vi "VI Tree.vi"   [LabVIEW 2011, in "Fluke 5XXX Series Multicalibrators.lvlib"]
doc: "This is the instrument driver for the following instruments FLUKE 5500A, 5520A, 5700A, 5720A and 57LFC including their options:\n\n 5725A ... Auxiliary amplifier\n SC300 ... 300 MHz Oscilloscope Calibration\n SC600 ... 600 MHz Oscilloscope Calibration\n SC1100 ... 1.1 GHz Oscilloscope Calibration\n 700P ... Pressure modules\n 5700A_03 ... Wideband AC Voltage\n\nThe VI Tree displays all the user-callable VIs of the instrument driver in an organized table."
uses:
  Fluke 5XXX Series Multicalibrators.lvlib
panel:
  # "© 2005 National Instruments.  ALL RIGHTS RESERVED."
  # "SEE DIAGRAM\nFOR VI TREE."
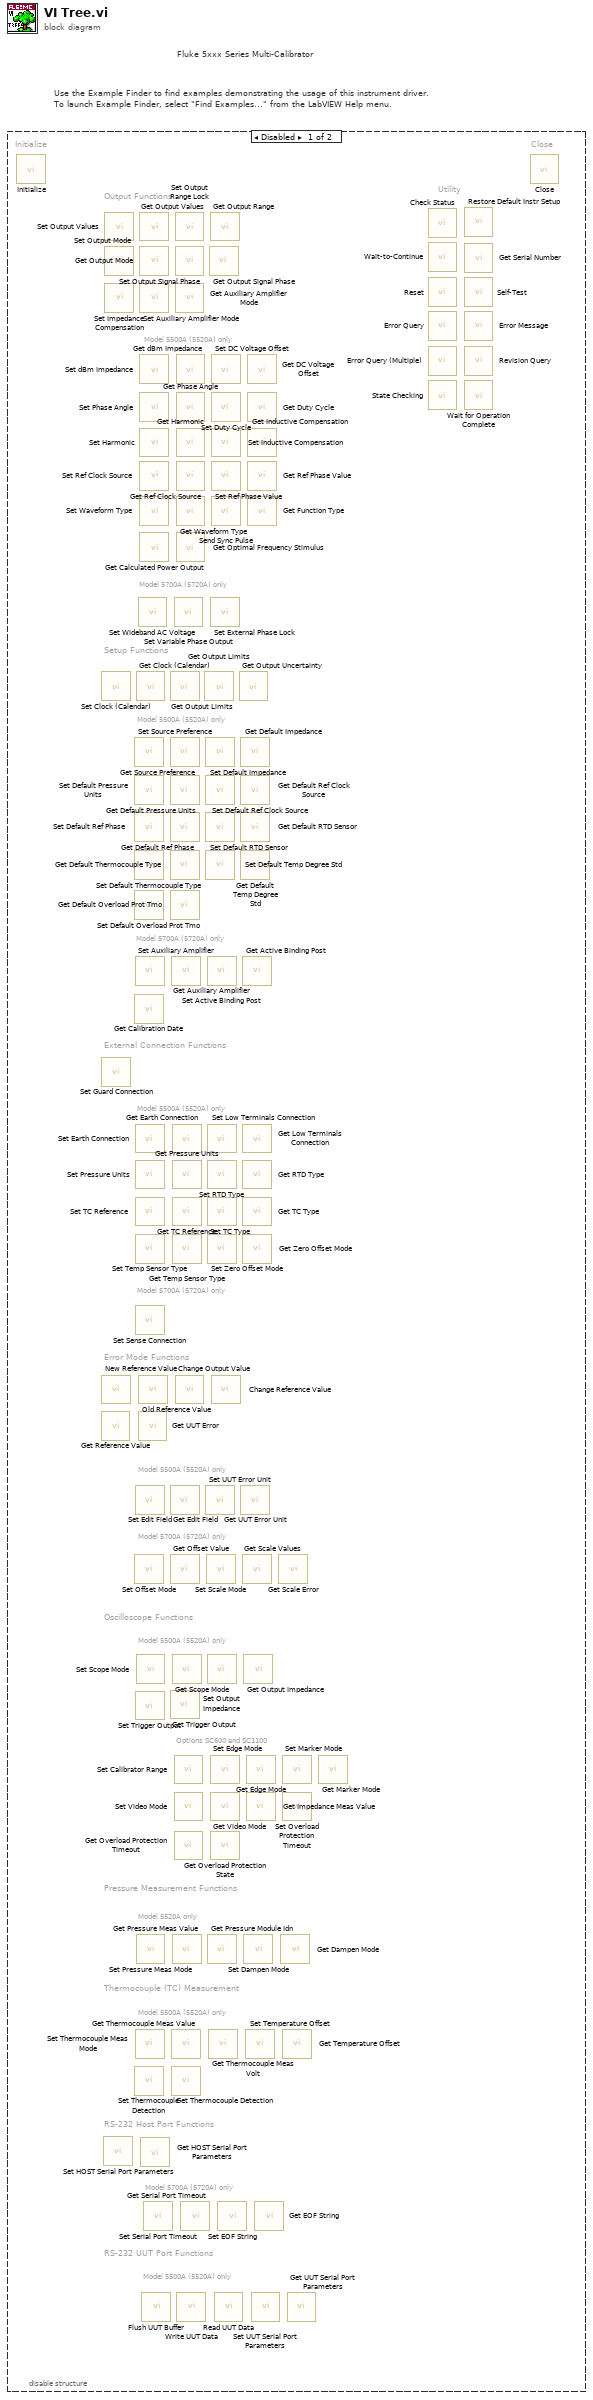
[diagram p0: block diagram]
diagram:
  # "Fluke 5xxx Series Multi-Calibrator"
  # "Use the Example Finder to find examples demonstrating the usage of this instrument driver.\nTo launch Example Finder, select \"Find Examples...\" from the LabVIEW Help menu."
  n1 = disable-structure shown="Disabled" {
    frame Disabled {
      # "Model 5500A (5520A) only"
      # "RS-232 UUT Port Functions"
      # "Model 5700A (5720A) only"
      # "RS-232 Host Port Functions"
      # "Model 5500A (5520A) only"
      # "Thermocouple (TC) Measurement"
      # "Model 5520A only"
      # "Pressure Measurement Functions"
      # "Options SC600 and SC1100"
      # "Model 5500A (5520A) only"
      # "Oscilloscope Functions"
      # "Model 5700A (5720A) only"
      # "Model 5500A (5520A) only"
      # "Error Mode Functions"
      # "Model 5700A (5720A) only"
      # "Model 5500A (5520A) only"
      # "External Connection Functions"
      # "Model 5700A (5720A) only"
      # "Model 5500A (5520A) only"
      # "Setup Functions"
      # "Model 5700A (5720A) only"
      # "Model 5500A (5520A) only"
      # "Output Functions"
      # "Utility"
      # "Close"
      # "Initialize"
      n2 = call "Initialize.vi"() -> ()  [unwired: 14 in, 2 out]
      n3 = call "Get Reference Value.vi"() -> ()  [unwired: 9 in, 3 out]
      n4 = call "Set Clock (Calendar).vi"() -> ()  [unwired: 14 in, 2 out]
      n5 = call "Set Guard Connection.vi"() -> ()  [unwired: 10 in, 2 out]
      n6 = call "New Reference Value.vi"() -> ()  [unwired: 10 in, 2 out]
      n7 = call "Set HOST Serial Port Parameters.vi"() -> ()  [unwired: 14 in, 2 out]
      n8 = call "Set Output Values.vi"() -> ()  [unwired: 10 in, 2 out]
      n9 = call "Set Output Mode.vi"() -> ()  [unwired: 10 in, 2 out]
      n10 = call "Set Impedance Compensation.vi"() -> ()  [unwired: 10 in, 2 out]
      n11 = call "Set Source Preference.vi"() -> ()  [unwired: 10 in, 2 out]
      n12 = call "Set Default Pressure Units.vi"() -> ()  [unwired: 10 in, 2 out]
      n13 = call "Set Default Ref Phase.vi"() -> ()  [unwired: 10 in, 2 out]
      n14 = call "Set Default Thermocouple Type.vi"() -> ()  [unwired: 10 in, 2 out]
      n15 = call "Set Default Overload Prot Tmo.vi"() -> ()  [unwired: 10 in, 2 out]
      n16 = call "Get Calibration Date.vi"() -> ()  [unwired: 7 in, 5 out]
      n17 = call "Set Offset Mode.vi"() -> ()  [unwired: 10 in, 2 out]
      n18 = call "Set Thermocouple Detection.vi"() -> ()  [unwired: 10 in, 2 out]
      n19 = call "Set Auxiliary Amplifier.vi"() -> ()  [unwired: 10 in, 2 out]
      n20 = call "Set Earth Connection.vi"() -> ()  [unwired: 10 in, 2 out]
      n21 = call "Set Pressure Units.vi"() -> ()  [unwired: 10 in, 2 out]
      n22 = call "Set TC Reference.vi"() -> ()  [unwired: 10 in, 2 out]
      n23 = call "Set Temp Sensor Type.vi"() -> ()  [unwired: 10 in, 2 out]
      n24 = call "Set Sense Connection.vi"() -> ()  [unwired: 10 in, 2 out]
      n25 = call "Set Edit Field.vi"() -> ()  [unwired: 10 in, 2 out]
      n26 = call "Set Trigger Output.vi"() -> ()  [unwired: 10 in, 2 out]
      n27 = call "Set Thermocouple Meas Mode.vi"() -> ()  [unwired: 10 in, 2 out]
      n28 = call "Get Clock (Calendar).vi"() -> ()  [unwired: 8 in, 8 out]
      n29 = call "Set Scope Mode.vi"() -> ()  [unwired: 10 in, 2 out]
      n30 = call "Set Pressure Meas Mode.vi"() -> ()  [unwired: 10 in, 2 out]
      n31 = call "Set Wideband AC Voltage.vi"() -> ()  [unwired: 10 in, 2 out]
      n32 = call "Get UUT Error.vi"() -> ()  [unwired: 8 in, 4 out]
      n33 = call "Old Reference Value.vi"() -> ()  [unwired: 10 in, 2 out]
      n34 = call "Get Output Values.vi"() -> ()  [unwired: 9 in, 7 out]
      n35 = call "Get Output Mode.vi"() -> ()  [unwired: 9 in, 3 out]
      n36 = call "Set Auxiliary Amplifier Mode.vi"() -> ()  [unwired: 10 in, 2 out]
      n37 = call "Set dBm Impedance.vi"() -> ()  [unwired: 10 in, 2 out]
      n38 = call "Set Phase Angle.vi"() -> ()  [unwired: 10 in, 2 out]
      n39 = call "Set Harmonic.vi"() -> ()  [unwired: 10 in, 2 out]
      n40 = call "Set Ref Clock Source.vi"() -> ()  [unwired: 10 in, 2 out]
      n41 = call "Set Waveform Type.vi"() -> ()  [unwired: 10 in, 2 out]
      n42 = call "Get Calculated Power Output.vi"() -> ()  [unwired: 9 in, 3 out]
      n43 = call "Get HOST Serial Port Parameters.vi"() -> ()  [unwired: 7 in, 9 out]
      n44 = call "Flush UUT Buffer.vi"() -> ()  [unwired: 10 in, 2 out]
      n45 = call "Set Serial Port Timeout.vi"() -> ()  [unwired: 10 in, 2 out]
      n46 = call "Get Output Limits.vi"() -> ()  [unwired: 8 in, 4 out]
      n47 = call "Get Source Preference.vi"() -> ()  [unwired: 9 in, 3 out]
      n48 = call "Get Default Pressure Units.vi"() -> ()  [unwired: 9 in, 3 out]
      n49 = call "Get Default Ref Phase.vi"() -> ()  [unwired: 9 in, 3 out]
      n50 = call "Get Default Thermocouple Type.vi"() -> ()  [unwired: 9 in, 3 out]
      n51 = call "Get Default Overload Prot Tmo.vi"() -> ()  [unwired: 9 in, 3 out]
      n52 = call "Get Edit Field.vi"() -> ()  [unwired: 9 in, 3 out]
      n53 = call "Get Offset Value.vi"() -> ()  [unwired: 8 in, 4 out]
      n54 = call "Get Trigger Output.vi"() -> ()  [unwired: 9 in, 3 out]
      n55 = call "Get Auxiliary Amplifier.vi"() -> ()  [unwired: 8 in, 4 out]
      n56 = call "Get Thermocouple Meas Value.vi"() -> ()  [unwired: 8 in, 4 out]
      n57 = call "Get Thermocouple Detection.vi"() -> ()  [unwired: 9 in, 3 out]
      n58 = call "Get Earth Connection.vi"() -> ()  [unwired: 9 in, 3 out]
      n59 = call "Get Pressure Units.vi"() -> ()  [unwired: 9 in, 3 out]
      n60 = call "Get TC Reference.vi"() -> ()  [unwired: 7 in, 5 out]
      n61 = call "Get Temp Sensor Type.vi"() -> ()  [unwired: 9 in, 3 out]
      n62 = call "Get Scope Mode.vi"() -> ()  [unwired: 9 in, 3 out]
      n63 = call "Get Pressure Meas Value.vi"() -> ()  [unwired: 8 in, 4 out]
      n64 = call "Set Variable Phase Output.vi"() -> ()  [unwired: 10 in, 2 out]
      n65 = call "Set Calibrator Range.vi"() -> ()  [unwired: 10 in, 2 out]
      n66 = call "Set Video Mode.vi"() -> ()  [unwired: 10 in, 2 out]
      n67 = call "Get Overload Protection Timeout.vi"() -> ()  [unwired: 9 in, 3 out]
      n68 = call "Set Output Range Lock.vi"() -> ()  [unwired: 10 in, 2 out]
      n69 = call "Set Output Signal Phase.vi"() -> ()  [unwired: 10 in, 2 out]
      n70 = call "Get Auxiliary Amplifier Mode.vi"() -> ()  [unwired: 9 in, 3 out]
      n71 = call "Change Output Value.vi"() -> ()  [unwired: 10 in, 2 out]
      n72 = call "Get dBm Impedance.vi"() -> ()  [unwired: 9 in, 3 out]
      n73 = call "Get Phase Angle.vi"() -> ()  [unwired: 8 in, 4 out]
      n74 = call "Get Harmonic.vi"() -> ()  [unwired: 8 in, 4 out]
      n75 = call "Get Ref Clock Source.vi"() -> ()  [unwired: 9 in, 3 out]
      n76 = call "Get Waveform Type.vi"() -> ()  [unwired: 8 in, 4 out]
      n77 = call "Get Optimal Frequency Stimulus.vi"() -> ()  [unwired: 9 in, 3 out]
      n78 = call "Write UUT Data.vi"() -> ()  [unwired: 10 in, 2 out]
      n79 = call "Get Serial Port Timeout.vi"() -> ()  [unwired: 9 in, 3 out]
      n80 = call "Get Output Limits.vi"() -> ()  [unwired: 8 in, 4 out]
      n81 = call "Set Default Impedance.vi"() -> ()  [unwired: 10 in, 2 out]
      n82 = call "Set Default Ref Clock Source.vi"() -> ()  [unwired: 10 in, 2 out]
      n83 = call "Set Default RTD Sensor.vi"() -> ()  [unwired: 10 in, 2 out]
      n84 = call "Set Default Temp Degree Std.vi"() -> ()  [unwired: 10 in, 2 out]
      n85 = call "Set UUT Error Unit.vi"() -> ()  [unwired: 10 in, 2 out]
      n86 = call "Set Scale Mode.vi"() -> ()  [unwired: 10 in, 2 out]
      n87 = call "Set Active Binding Post.vi"() -> ()  [unwired: 10 in, 2 out]
      n88 = call "Set Low Terminals Connection.vi"() -> ()  [unwired: 10 in, 2 out]
      n89 = call "Set RTD Type.vi"() -> ()  [unwired: 10 in, 2 out]
      n90 = call "Set TC Type.vi"() -> ()  [unwired: 10 in, 2 out]
      n91 = call "Set Zero Offset Mode.vi"() -> ()  [unwired: 10 in, 2 out]
      n92 = call "Set Output Impedance.vi"() -> ()  [unwired: 10 in, 2 out]
      n93 = call "Get Pressure Module Idn.vi"() -> ()  [unwired: 7 in, 5 out]
      n94 = call "Get Thermocouple Meas Volt.vi"() -> ()  [unwired: 9 in, 3 out]
      n95 = call "Get Output Signal Phase.vi"() -> ()  [unwired: 9 in, 3 out]
      n96 = call "Get Output Range.vi"() -> ()  [unwired: 8 in, 4 out]
      n97 = call "Set External Phase Lock.vi"() -> ()  [unwired: 10 in, 2 out]
      n98 = call "Set Edge Mode.vi"() -> ()  [unwired: 10 in, 2 out]
      n99 = call "Get Video Mode.vi"() -> ()  [unwired: 8 in, 4 out]
      n100 = call "Get Overload Protection State.vi"() -> ()  [unwired: 9 in, 3 out]
      n101 = call "Set DC Voltage Offset.vi"() -> ()  [unwired: 10 in, 2 out]
      n102 = call "Set Duty Cycle.vi"() -> ()  [unwired: 10 in, 2 out]
      n103 = call "Set Inductive Compensation.vi"() -> ()  [unwired: 10 in, 2 out]
      n104 = call "Set Ref Phase Value.vi"() -> ()  [unwired: 10 in, 2 out]
      n105 = call "Send Sync Pulse.vi"() -> ()  [unwired: 10 in, 2 out]
      n106 = call "Change Reference Value.vi"() -> ()  [unwired: 10 in, 2 out]
      n107 = call "Read UUT Data.vi"() -> ()  [unwired: 8 in, 4 out]
      n108 = call "Set EOF String.vi"() -> ()  [unwired: 10 in, 2 out]
      n109 = call "Get Output Uncertainty.vi"() -> ()  [unwired: 7 in, 5 out]
      n110 = call "Get Default Impedance.vi"() -> ()  [unwired: 9 in, 3 out]
      n111 = call "Get Default Ref Clock Source.vi"() -> ()  [unwired: 9 in, 3 out]
      n112 = call "Get Default RTD Sensor.vi"() -> ()  [unwired: 9 in, 3 out]
      n113 = call "Get Default Temp Degree Std.vi"() -> ()  [unwired: 9 in, 3 out]
      n114 = call "Get UUT Error Unit.vi"() -> ()  [unwired: 9 in, 3 out]
      n115 = call "Get Active Binding Post.vi"() -> ()  [unwired: 9 in, 3 out]
      n116 = call "Get Low Terminals Connection.vi"() -> ()  [unwired: 9 in, 3 out]
      n117 = call "Get RTD Type.vi"() -> ()  [unwired: 9 in, 3 out]
      n118 = call "Get TC Type.vi"() -> ()  [unwired: 9 in, 3 out]
      n119 = call "Get Zero Offset Mode.vi"() -> ()  [unwired: 7 in, 5 out]
      n120 = call "Get Scale Values.vi"() -> ()  [unwired: 7 in, 5 out]
      n121 = call "Get Output Impedance.vi"() -> ()  [unwired: 9 in, 3 out]
      n122 = call "Set Dampen Mode.vi"() -> ()  [unwired: 10 in, 2 out]
      n123 = call "Set Temperature Offset.vi"() -> ()  [unwired: 10 in, 2 out]
      n124 = call "Get Edge Mode.vi"() -> ()  [unwired: 9 in, 3 out]
      n125 = call "Get Impedance Meas Value.vi"() -> ()  [unwired: 8 in, 4 out]
      n126 = call "Get DC Voltage Offset.vi"() -> ()  [unwired: 9 in, 3 out]
      n127 = call "Get Duty Cycle.vi"() -> ()  [unwired: 9 in, 3 out]
      n128 = call "Get Inductive Compensation.vi"() -> ()  [unwired: 9 in, 3 out]
      n129 = call "Get Ref Phase Value.vi"() -> ()  [unwired: 9 in, 3 out]
      n130 = call "Get Function Type.vi"() -> ()  [unwired: 9 in, 3 out]
      n131 = call "Set UUT Serial Port Parameters.vi"() -> ()  [unwired: 14 in, 2 out]
      n132 = call "Get EOF String.vi"() -> ()  [unwired: 8 in, 4 out]
      n133 = call "Get Scale Error.vi"() -> ()  [unwired: 8 in, 4 out]
      n134 = call "Get Dampen Mode.vi"() -> ()  [unwired: 9 in, 3 out]
      n135 = call "Set Marker Mode.vi"() -> ()  [unwired: 10 in, 2 out]
      n136 = call "Set Overload Protection Timeout.vi"() -> ()  [unwired: 10 in, 2 out]
      n137 = call "Get Temperature Offset.vi"() -> ()  [unwired: 8 in, 4 out]
      n138 = call "Get UUT Serial Port Parameters.vi"() -> ()  [unwired: 9 in, 7 out]
      n139 = call "Get Marker Mode.vi"() -> ()  [unwired: 9 in, 3 out]
      n140 = call "Check Status.vi"() -> ()  [unwired: 14 in, 2 out]
      n141 = call "Wait-to-Continue.vi"() -> ()  [unwired: 10 in, 2 out]
      n142 = call "Reset.vi"() -> ()  [unwired: 14 in, 2 out]
      n143 = call "Error Query.vi"() -> ()  [unwired: 12 in, 4 out]
      n144 = call "Error Query (Multiple).vi"() -> ()  [unwired: 12 in, 4 out]
      n145 = call "State Checking.vi"() -> ()  [unwired: 10 in, 2 out]
      n146 = call "Restore Default Instr Setup.vi"() -> ()  [unwired: 10 in, 2 out]
      n147 = call "Get Serial Number.vi"() -> ()  [unwired: 9 in, 3 out]
      n148 = call "Self-Test.vi"() -> ()  [unwired: 12 in, 4 out]
      n149 = call "Error Message.vi"() -> ()  [unwired: 11 in, 5 out]
      n150 = call "Revision Query.vi"() -> ()  [unwired: 12 in, 4 out]
      n151 = call "Wait for Operation Complete.vi"() -> ()  [unwired: 10 in, 2 out]
      n152 = call "Close.vi"() -> ()  [unwired: 15 in, 1 out]
    }
    frame Enabled {
    }
  }
